vi "SLL DE 1D Array Moving Average.vi"(7 "Old Points":dbl[](array[numeric]), 9 "MvgAvg WindowSize":i32=20, 11 "Input Array":dbl[](array[numeric])) -> (3 "Output Array":dbl[](array[numeric]))   [LabVIEW 2013]
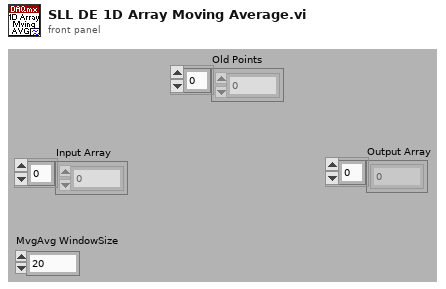
[diagram p1: front panel]
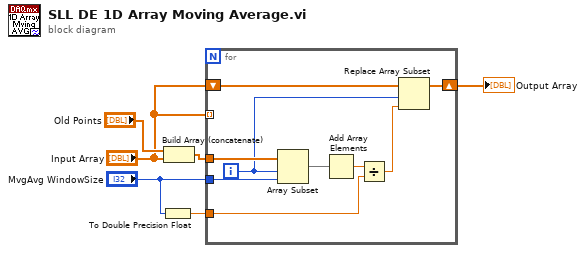
[diagram p0: block diagram]
diagram:
  n1 = To Double Precision Float(number="MvgAvg WindowSize") -> (double precision float=w6:dbl)
  n2 = Build Array (concatenate)("Old Points", "Input Array") -> (w3:dbl[])
  n3 = for {
    shift-right: [w12] -> w4
    shift-left: "Input Array" -> [w13]
    tunnel: w3 -> [w14]
    tunnel: "MvgAvg WindowSize" -> [w15]
    tunnel: w6 -> [w9]
    tunnel: "Input Array" -> [_] mode=indexing
    i -> [w11]
    n4 = Array Subset(array=w14, index=w11, length=w15) -> (w8:dbl[])
    n5 = Add Array Elements(numeric array=w8) -> (sum=w10:dbl)
    n6 = Divide(x=w10, y=w9) -> (x/y=w7:dbl)
    n7 = Replace Array Subset(array=w13, new element=w7, index=w11) -> (w12:dbl[])
  }
  "Output Array" <- w4
